vi "SOUR_POW_CORR_COLL_BSEN_SEL.vi"(0 "VISA IN":refnum<visa-resource-name>, 5 "error in":errorcluster, 7 "Channel":i32) -> (14 "VISA Out":refnum<visa-resource-name>, 16 "Data":string, 19 "error out":errorcluster)   [LabVIEW 2018, in "PNA-X.lvlib"]
doc: "SOURce:POWer:CORRection:COLLect:BSENsor:SELect? <Frequency> \nReturns a boolean 1 or 0 (true or false) indicating whether the sensor is to be \nused at the specified frequency. \nIf frequency checking is OFF, then the <Frequency> parameter is ignored. The \nquery returns if the sensor is selected for ALL frequencies. \nReturn Type Numeric \nDefault Not Applicable \nSOURce<cnum>:POWer:CORRection:COLLect:TABLe:DATA <data> \n1843\n\n(Read-Write) Read or write data into the selected table. Use \nSOUR:POW:CORR:COLL:TABL:SELect to select a table. \nIf the selected table is a power sensor table, the data is interpreted as cal factors in percent. \nIf the loss table is selected, the data is interpreted as loss in dB. \nParameters \n<cnum> Any existing channel number. If unspecified, value is set to 1 \n<data> Data to write into the selected table. \nExamples SOURce:POWer:CORRection:COLLect:TABLe:DATA 0.12, 0.34, 0.56 \nQuery Syntax SOURce<cnum>:POWer:CORRection:COLLect:TABLe:DATA? \nIf the selected table is currently empty, no data is returned. \nReturn Type Numeric - one number per table segment. \nDefault Not Applicable \nSOURce<cnum>:POWer:CORRection:COLLect:TABLe:FREQuency <data> \n(Read-Write) Read or write frequency values for the selected table (cal factor table for a power sensor, \nor the loss compensation table). \nParameters \n<cnum> Any existing channel number. If unspecified, value is set to 1 \n<data> Frequency data to write into the selected table. \nExamples SOURce:POWer:CORRection:COLLect:TABLe:FREQuency 10E6, 1.5E9, 9E9 \nQuery Syntax SOURce<cnum>:POWer:CORRection:COLLect:TABLe:FREQuency? \nIf the selected table is currently empty, no data is returned. \nReturn Type Numeric - one number per table segment \nDefault Not Applicable \nSOURce<cnum>:POWer:CORRection:COLLect:TABLe:LOSS[:STATe] <ON | OFF> \n1844\n\n(Read-Write) Indicates whether or not to adjust the power readings using the values in the loss table \nduring a source power cal sweep. \nParameters \n<cnum> Any existing channel number. If unspecified, value is set to 1 \n<ON|OFF> ON (or 1) - turns use of the loss table ON. \nOFF (or 0) - turns use of the loss table OFF. \nExamples SOUR:POW:CORR:COLL:TABL:LOSS ON \nsource1:power2:correction:collect:table:loss:state off \nQuery Syntax SOURce:POWer:CORRection:COLLect:TABLe:LOSS[:STATe]? \nReturn Type Boolean (1 = ON, 0 = OFF) \nDefault OFF (0) \nSOURce<cnum>:POWer:CORRection:COLLect:TABLe:POINts? \n(Read-only) Returns the number of segments that are currently in the selected table. \nParameters \n<cnum> Any existing channel number. If unspecified, value is set to 1 \nExamples SOUR:POW:CORR:COLL:TABL:POIN? \nsource1:power2:correction:collect:table:points? \nReturn Type Numeric \nDefault 0 \nSOURce<cnum>:POWer:CORRection:COLLect:TABLe[:SELect] <char> \n1845\n\n(Read-Write) Selects which table you want to write to or read from. Read or write using"
uses:
  PNA-X.lvlib
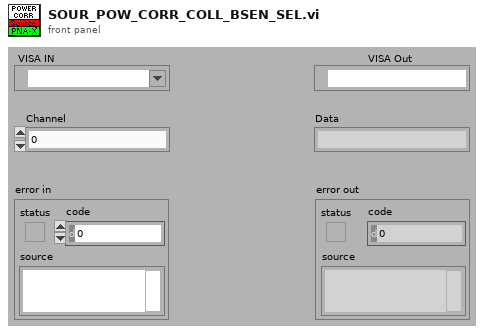
[diagram p1: front panel]
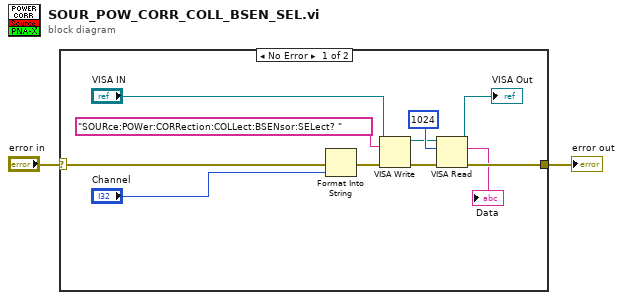
[diagram p0: block diagram]
diagram:
  n1 = case shown="No Error" "error in" {
    selector: "error in" -> [w13 w14]
    tunnel: [w7 w14] -> w1
    frame No Error {
      n2 = Format Into String(error in=w13, "Channel") -> (error out=w12:errorcluster)  [unwired: 2 in, 1 out]
      n3 = VISA Write(VISA resource name="VISA IN", write buffer="SOURce:POWer:CORRection:COLLect:BSENsor:SELect? " ("Cmdline"), error in (no error)=w12) -> (VISA resource name out=w8:refnum<visa-resource-name>, error out=w10:errorcluster)  [unwired: 1 out]
      n4 = VISA Read(VISA resource name=w8, byte count=1024, error in (no error)=w10) -> (VISA resource name out=→"VISA Out":refnum<visa-resource-name>, read buffer=→"Data":string, error out=w7:errorcluster)  [unwired: 1 out]
    }
    frame Error {
    }
  }
  "error out" <- w1
